vi "SGDA-Write To Signal Bank.vi"(4 "error in (no error)":errorcluster, 5 "Input array":dbl[][](array[numeric]) format="%.2f", 6 "Active AO Array":u16[](array[numeric]), 7 "timeout (ms)":i32=5000) -> (0 "error out":errorcluster={"status"=FALSE, "code"=0, "source"="."})   [LabVIEW 2015]
uses:
  SGDA-Globals.vi
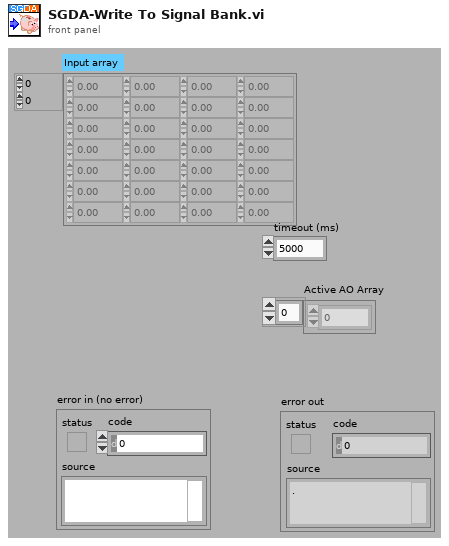
[diagram p1: front panel]
types:
  T1 = typedef "Hardware Destination.ctl" = enum16{"None", "PXI", "TDT", "NI", "TDTSIM"}
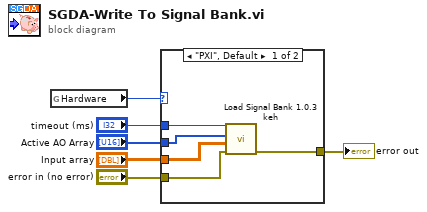
[diagram p0: block diagram]
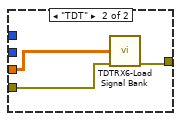
[diagram p2: hidden frame]
diagram:
  n1 = global read "SGDA-Globals.vi" "Hardware"() -> (w6:T1)
  n2 = case shown="\"PXI\", Default" w6 {
    tunnel: "timeout (ms)" -> [w11 _]
    tunnel: "Active AO Array" -> [w10 _]
    tunnel: "Input array" -> [w9 w12]
    tunnel: "error in (no error)" -> [w8 w13]
    tunnel: [w7 w14] -> w1
    frame "PXI", Default {
      n3 = call "Load Signal Bank 1.0.3 keh.vi"("error in (no error)"=w8, "Input array"=w9, "Active AO Array"=w10, "timeout (ms)"=w11) -> ("error out"=w7:errorcluster)  [unwired: 5 in, 2 out]
    }
    frame "TDT" {
      n4 = call "TDTRX6-Load Signal Bank.vi"("Output array"=w12, "error in (no error)"=w13) -> ("error out"=w14:errorcluster)  [unwired: 13 in]
    }
  }
  "error out" <- w1
